vi "首页.vi"() -> ()   [LabVIEW 2016]
uses:
  <vilib>/Utility/miscctls.llb/LVPointTypeDef.ctl
  <vilib>/Utility/sysdir.llb/System Directory Type.ctl
  <vilib>/addons/database/_DB Variant To Data/Database Variant To Data.xnode
  PLC/PLC.lvlib
panel:
  out "小项目框 10":T1(xcontrol)
  out "小项目框 9":T1(xcontrol)
  out "小项目框 4":T1(xcontrol)
  out "小项目框 3":T1(xcontrol)
  out "小项目框 2":T1(xcontrol)
  out "小项目框 8":T1(xcontrol)
  out "小项目框 7":T1(xcontrol)
  out "小项目框 6":T1(xcontrol)
  out "小项目框 5":T1(xcontrol)
  out "小项目框":T1(xcontrol)
  out "湿度":string="75.5 %"
  out "室温":string="25.8 ℃"
  # "湿度:"
  # "室温:"
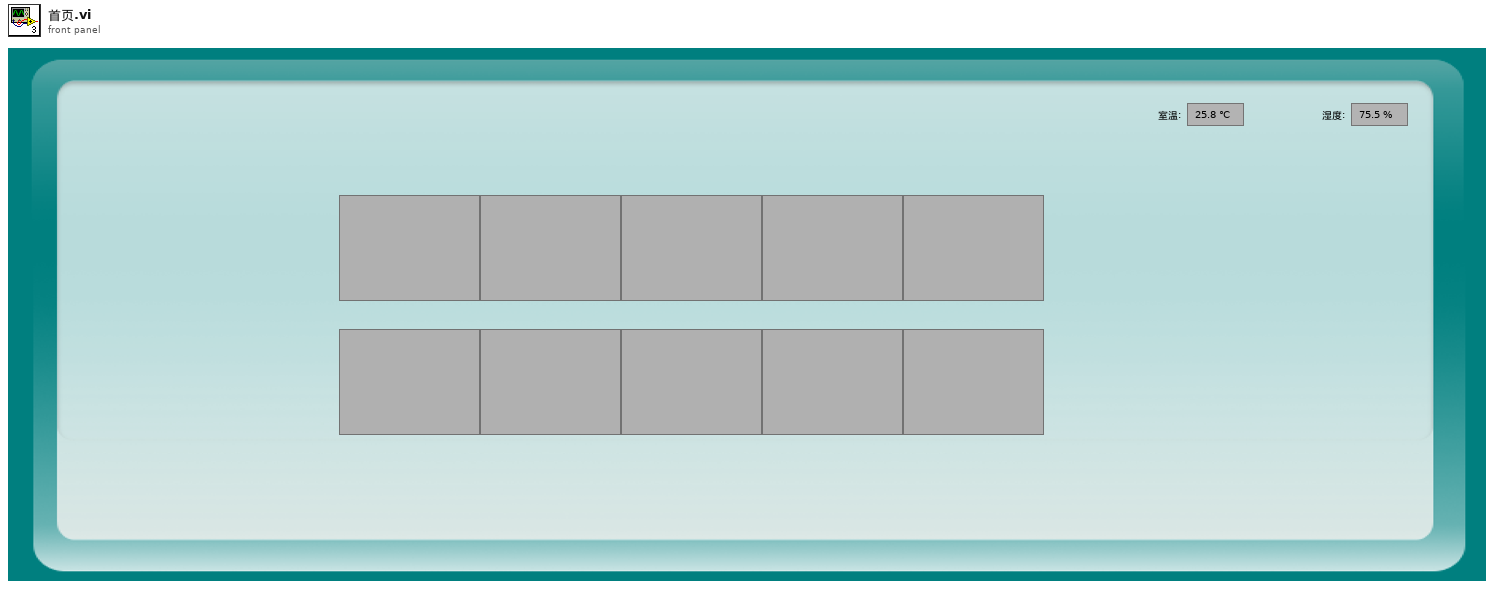
[diagram p1: front panel]
types:
  T1 = cluster{"中文项目名称":string, "英文项目名称":string, "单位":string, "浓度值":sgl, "精度":sgl}
  T2 = typedef "System Directory Type.ctl" = i32
  T3 = typedef "LVPointTypeDef.ctl" = cluster{"Horizontal":i16, "Vertical":i16}
  T4 = cluster{"AD0":sgl, "AD1":sgl, "AD2":sgl, "AD3":sgl, "AD4":sgl, "AD5":sgl}
  T5 = typedef "LVDateTimeRec.ctl" = cluster{"秒数的小数部分":dbl, "秒":i32, "分":i32, "时":i32, "日":i32, "月":i32, "年":i32, "天数（周）":i32, "天数（年）":i32, "DST":i32}
  T6 = cluster{"seconds since 1Jan1904":timestamp, "AD0":sgl, "单位":u16}
  T7 = cluster{"seconds since 1Jan1904":timestamp, "AD1":sgl, "单位":u16}
  T8 = cluster{"时间标识":timestamp, "监测值":sgl, "单位":string}
  T9 = cluster{"中文项目名称":string, "英文项目名称":string, "单位":string, "浓度值":sgl, "浓度值 2":sgl}
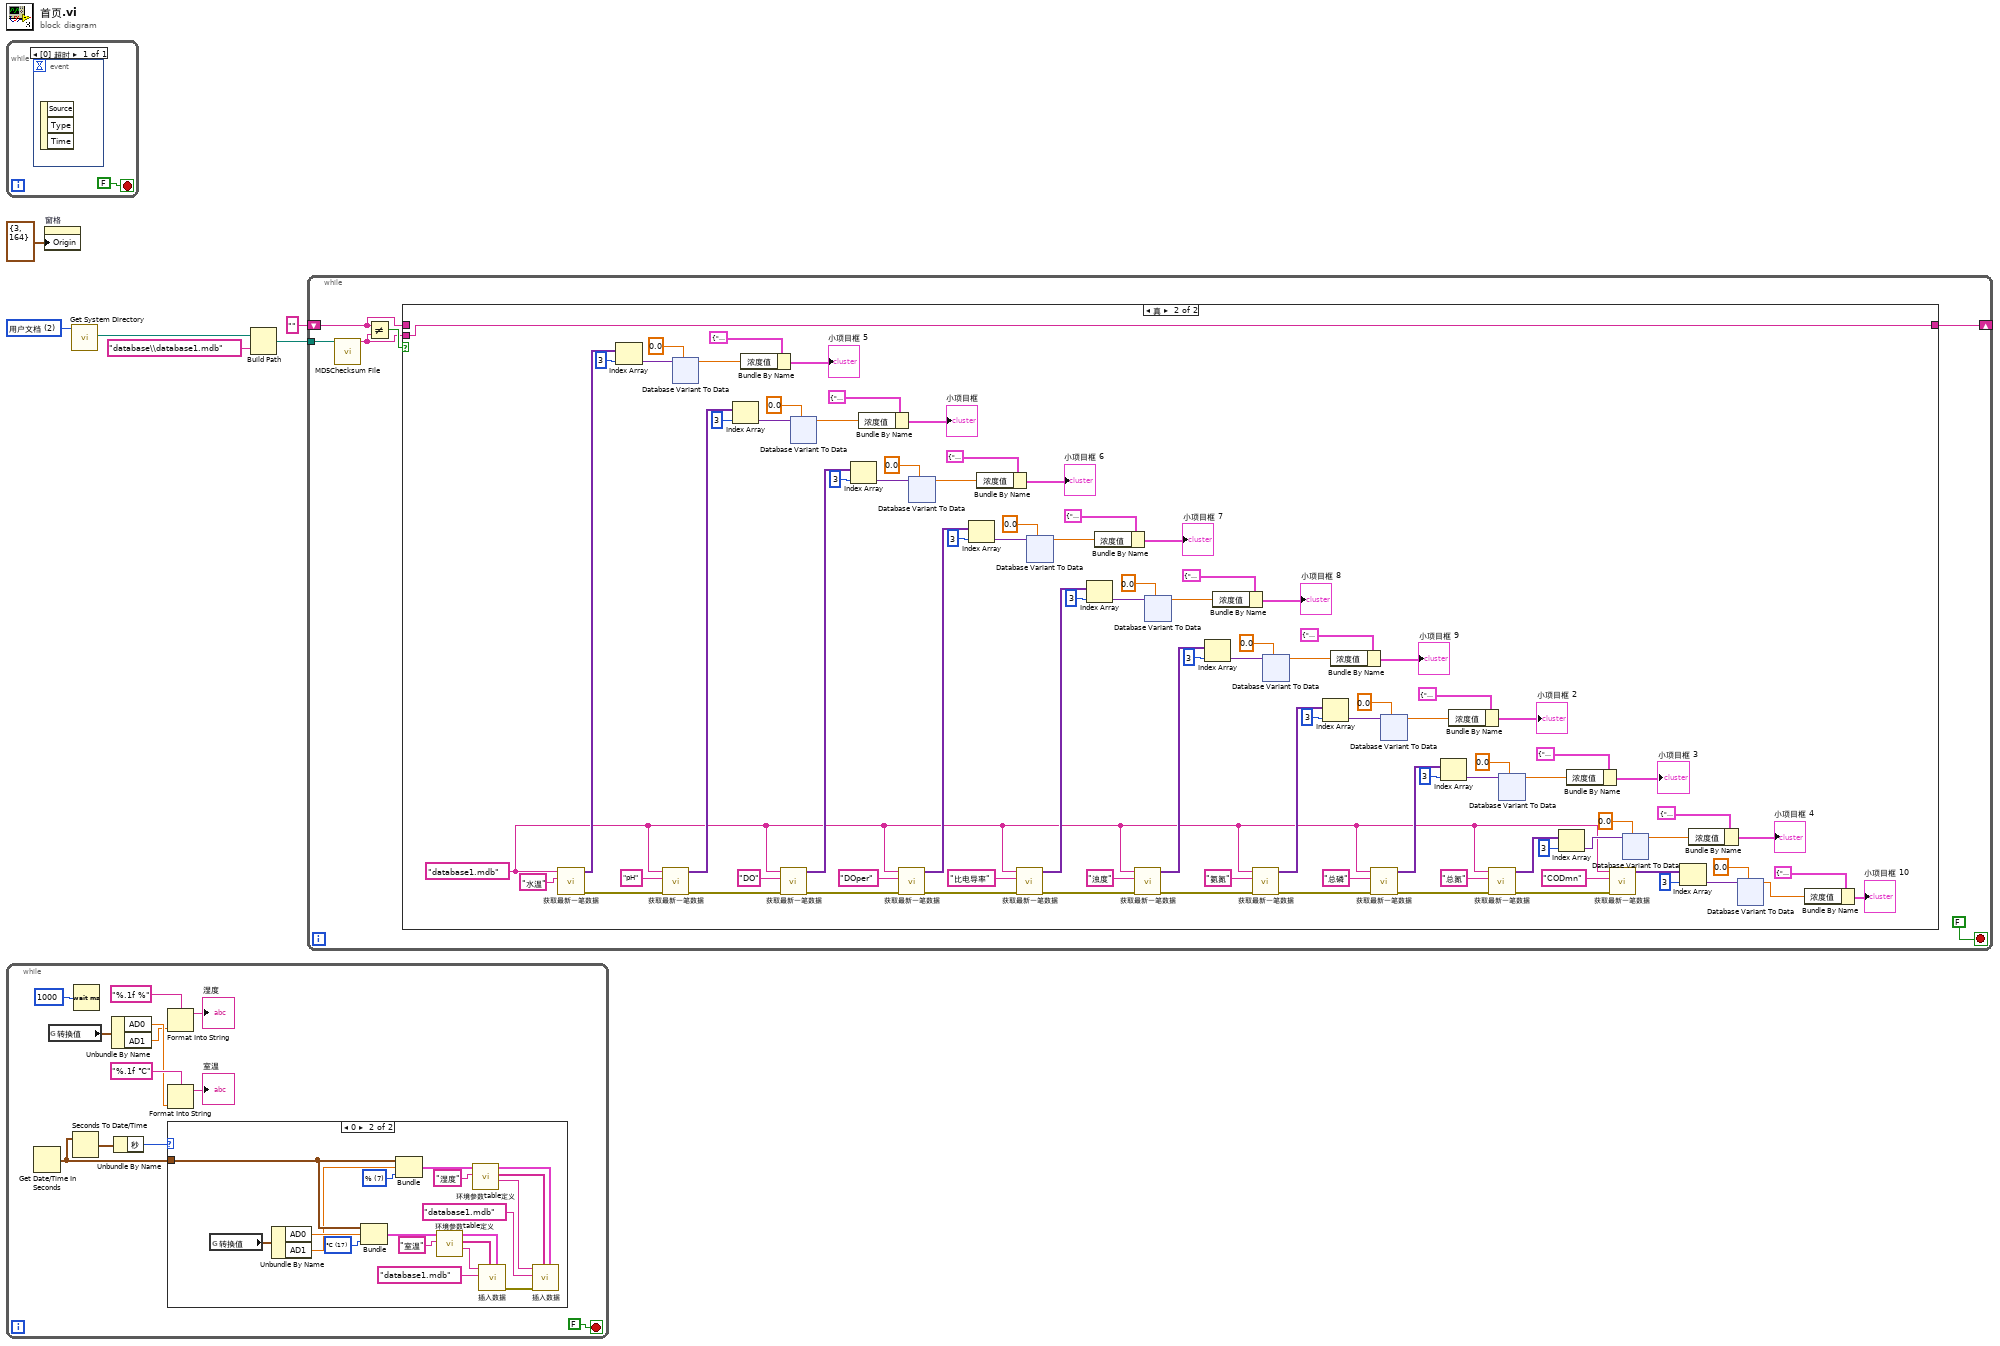
[diagram p0: block diagram]
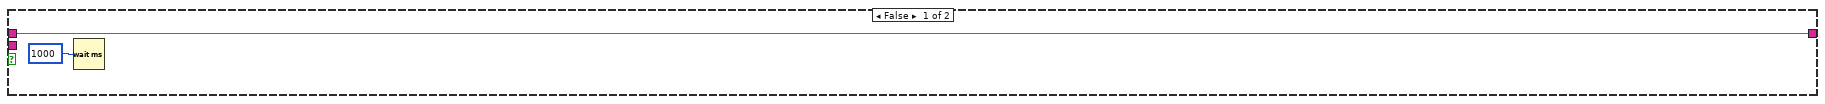
[diagram p2: hidden frame]
diagram:
  w5 = T2 2 items=["用户目录"=0, "用户桌面"=1, "用户文档"=2, "用户应用程序数据"=3, "用户设置"=4, "用户临时目录"=5, "公共文档"=6, "公共应用程序数据"=7, "公共设置"=8, "公共缓存"=13, "系统核心库"=9, "系统安装库"=10, "应用程序文件"=11, "启动盘根目录"=12] ("system directory type")
  n1 = while {
    stop <- FALSE stop-if-true
    n2 = event shown="[0] 超时" {
      selector: _ -> [_]
      dyn-events: _ -> [_]
      timeout: _ -> [_]
      event Timeout {
        n3 = event-data() -> ()  [unwired: 1 in, 3 out]
      }
    }
  }
  n4 = while {
    stop <- FALSE stop-if-true
    n5 = Get Date/Time In Seconds() -> (seconds since 1Jan1904=w10:timestamp)
    n6 = global read "采配水全局变量.vi" "转换值"() -> (w17:T4)
    n7 = Seconds To Date/Time(time stamp (now)=w10) -> (date time rec=w9:T5)  [unwired: 1 in]
    n8 = Wait (ms)(milliseconds to wait=u32 1000 ("等待时间（毫秒）")) -> ()  [unwired: 1 out]
    n9 = Unbundle By Name(w17) -> ("AD0"=w12:sgl, "AD1"=w11:sgl)
    n10 = Unbundle By Name(w9) -> ("秒"=w8:i32)
    n11 = Format Into String(format string="%.1f %" ("格式字符串"), w11) -> (resulting string=→"湿度":string)  [unwired: 2 in, 1 out]
    n12 = Format Into String(format string="%.1f ℃" ("格式字符串"), w12) -> (resulting string=→"室温":string)  [unwired: 2 in, 1 out]
    n13 = case shown="0" w8 {
      tunnel: w10 -> [_ w25]
      frame Default {
      }
      frame 0 {
        w23 = u16 7 items=["ug/L", "mg/L", "ppm", "mg/m3", "cm", "ppb", "ug/m3", "%", "nmol/mol", "umol/mol", "MPN/L", "MPN/100ml", "ng/m3", "NTU", "无量纲", "ms/cm", "us/cm", "℃"] ("单位")
        w26 = u16 17 items=["ug/L", "mg/L", "ppm", "mg/m3", "cm", "ppb", "ug/m3", "%", "nmol/mol", "umol/mol", "MPN/L", "MPN/100ml", "ng/m3", "NTU", "无量纲", "ms/cm", "us/cm", "℃"] ("单位")
        n14 = global read "采配水全局变量.vi" "转换值"() -> (w34:T4)
        n15 = Unbundle By Name(w34) -> ("AD0"=w28:sgl, "AD1"=w24:sgl)
        n16 = Bundle("seconds since 1Jan1904"=w25, "AD0"=w28, "单位"=w26) -> (w27:T6)  [unwired: 1 in]
        n17 = Bundle("seconds since 1Jan1904"=w25, "AD1"=w24, "单位"=w23) -> (w22:T7)  [unwired: 1 in]
        n18 = call "环境参数table定义.vi"("table 输入"="室温", "data"=w27) -> ("table 输出"=w35:string, "columns"=w36:string[], "data输出"=w37:T8)  [unwired: 7 in]
        n19 = call "环境参数table定义.vi"("table 输入"="湿度", "data"=w22) -> ("table 输出"=w33:string, "columns"=w32:string[], "data输出"=w31:T8)  [unwired: 7 in]
        n20 = call "插入数据.vi"("data"=w37, "columns"=w36, "database"="database1.mdb", "table"=w35) -> ("error out"=w29:errorcluster)  [unwired: 7 in]
        n21 = call "插入数据.vi"("data"=w31, "columns"=w32, "error in (no error)"=w29, "database"="database1.mdb", "table"=w33) -> ()  [unwired: 6 in, 1 out]
      }
    }
  }
  n22 = property on="窗格" class="Pane"("Origin"=T3 {"Horizontal"=3, "Vertical"=164} ("原点")) -> ()  [unwired: 2 in, 2 out]
  n23 = call <vilib>:"Get System Directory.vi"("system directory type"=w5) -> ("system directory"=w4:path)  [unwired: 10 in]
  n24 = Build Path(base path=w4, name or relative path="database\\database1.mdb" ("名称或相对路径")) -> (appended path=w2:path)
  n25 = while {
    tunnel: w2 -> [w44]
    shift-right: [w41] -> _
    shift-left: "" ("MD5 message-digest") -> [w40]
    stop <- FALSE stop-if-true
    n26 = call <vilib>:"MD5Checksum File.vi"("Path"=w44) -> ("MD5 message-digest"=w42:string)  [unwired: 9 in, 1 out]
    n27 = Not Equal?(x=w40, y=w42) -> (x != y?=w43:bool)
    n28 = case shown="真" w43 {
      tunnel: w42 -> [_ w137]
      tunnel: [w46 w137] -> w41
      tunnel: w40 -> [w46 _]
      frame False {
        n29 = Wait (ms)(milliseconds to wait=u32 1000 ("等待时间（毫秒）")) -> ()  [unwired: 1 out]
      }
      frame True {
        w55 = "database1.mdb" ("名称或相对路径")
        n30 = call "获取最新一笔数据.vi"("table"="水温", "database"=w55) -> ("error out"=w101:errorcluster, "子数组"=w67:variant[])  [unwired: 8 in]
        n31 = Index Array(array=w67, index=3 ("索引")) -> (element=w90:variant)
        n32 = call "获取最新一笔数据.vi"("error in (no error)"=w101, "table"="pH", "database"=w55) -> ("error out"=w100:errorcluster, "子数组"=w126:variant[])  [unwired: 7 in]
        n33 = xnode "Database Variant To Data"("database variant"=w90, "type"=0.0) -> ("data"=w92:dbl)  [unwired: 1 in, 1 out]
        n34 = Index Array(array=w126, index=3 ("索引")) -> (element=w109:variant)
        n35 = Bundle By Name(cluster=T9 {"中文项目名称"="水温", "英文项目名称"="T", "单位"="℃", "浓度值"=0.0, "浓度值 2"=2.0} ("小项目框 9"), "浓度值"=w92) -> (→"小项目框 5":T9)
        n36 = call "获取最新一笔数据.vi"("error in (no error)"=w100, "table"="DO", "database"=w55) -> ("error out"=w98:errorcluster, "子数组"=w66:variant[])  [unwired: 7 in]
        n37 = xnode "Database Variant To Data"("database variant"=w109, "type"=0.0) -> ("data"=w107:dbl)  [unwired: 1 in, 1 out]
        n38 = Index Array(array=w66, index=3 ("索引")) -> (element=w85:variant)
        n39 = Bundle By Name(cluster=T9 {"中文项目名称"="酸碱度", "英文项目名称"="pH", "单位"="", "浓度值"=0.0, "浓度值 2"=2.0} ("小项目框 9"), "浓度值"=w107) -> (→"小项目框":T9)
        n40 = call "获取最新一笔数据.vi"("error in (no error)"=w98, "table"="DOper", "database"=w55) -> ("error out"=w96:errorcluster, "子数组"=w65:variant[])  [unwired: 7 in]
        n41 = xnode "Database Variant To Data"("database variant"=w85, "type"=0.0) -> ("data"=w83:dbl)  [unwired: 1 in, 1 out]
        n42 = Index Array(array=w65, index=3 ("索引")) -> (element=w80:variant)
        n43 = Bundle By Name(cluster=T9 {"中文项目名称"="溶解氧", "英文项目名称"="DO", "单位"="mg/L", "浓度值"=0.0, "浓度值 2"=2.0} ("小项目框 9"), "浓度值"=w83) -> (→"小项目框 6":T9)
        n44 = call "获取最新一笔数据.vi"("error in (no error)"=w96, "table"="比电导率", "database"=w55) -> ("error out"=w94:errorcluster, "子数组"=w64:variant[])  [unwired: 7 in]
        n45 = xnode "Database Variant To Data"("database variant"=w80, "type"=0.0) -> ("data"=w82:dbl)  [unwired: 1 in, 1 out]
        n46 = Index Array(array=w64, index=3 ("索引")) -> (element=w75:variant)
        n47 = Bundle By Name(cluster=T9 {"中文项目名称"="溶解氧%", "英文项目名称"="DO%", "单位"="%", "浓度值"=0.0, "浓度值 2"=2.0} ("小项目框 9"), "浓度值"=w82) -> (→"小项目框 7":T9)
        n48 = call "获取最新一笔数据.vi"("error in (no error)"=w94, "table"="浊度", "database"=w55) -> ("error out"=w93:errorcluster, "子数组"=w63:variant[])  [unwired: 7 in]
        n49 = xnode "Database Variant To Data"("database variant"=w75, "type"=0.0) -> ("data"=w73:dbl)  [unwired: 1 in, 1 out]
        n50 = Index Array(array=w63, index=3 ("索引")) -> (element=w70:variant)
        n51 = Bundle By Name(cluster=T9 {"中文项目名称"="电导率", "英文项目名称"="Cond", "单位"="uS/cm", "浓度值"=0.0, "浓度值 2"=2.0} ("小项目框 9"), "浓度值"=w73) -> (→"小项目框 8":T9)
        n52 = call "获取最新一笔数据.vi"("error in (no error)"=w93, "table"="氨氮", "database"=w55) -> ("error out"=w135:errorcluster, "子数组"=w121:variant[])  [unwired: 7 in]
        n53 = xnode "Database Variant To Data"("database variant"=w70, "type"=0.0) -> ("data"=w72:dbl)  [unwired: 1 in, 1 out]
        n54 = Index Array(array=w121, index=3 ("索引")) -> (element=w115:variant)
        n55 = Bundle By Name(cluster=T9 {"中文项目名称"="浊度", "英文项目名称"="Turb", "单位"="NTU", "浓度值"=0.0, "浓度值 2"=2.0} ("小项目框 9"), "浓度值"=w72) -> (→"小项目框 9":T9)
        n56 = call "获取最新一笔数据.vi"("error in (no error)"=w135, "table"="总磷", "database"=w55) -> ("error out"=w103:errorcluster, "子数组"=w116:variant[])  [unwired: 7 in]
        n57 = xnode "Database Variant To Data"("database variant"=w115, "type"=0.0) -> ("data"=w113:dbl)  [unwired: 1 in, 1 out]
        n58 = Index Array(array=w116, index=3 ("索引")) -> (element=w112:variant)
        n59 = Bundle By Name(cluster=T9 {"中文项目名称"="氨氮", "英文项目名称"="NH3-N", "单位"="mg/L", "浓度值"=0.0, "浓度值 2"=3.0} ("小项目框 9"), "浓度值"=w113) -> (→"小项目框 2":T9)
        n60 = call "获取最新一笔数据.vi"("error in (no error)"=w103, "table"="总氮", "database"=w55) -> ("error out"=w56:errorcluster, "子数组"=w129:variant[])  [unwired: 7 in]
        n61 = xnode "Database Variant To Data"("database variant"=w112, "type"=0.0) -> ("data"=w110:dbl)  [unwired: 1 in, 1 out]
        n62 = Index Array(array=w129, index=3 ("索引")) -> (element=w106:variant)
        n63 = Bundle By Name(cluster=T9 {"中文项目名称"="总磷", "英文项目名称"="TP", "单位"="mg/L", "浓度值"=0.0, "浓度值 2"=3.0} ("小项目框 9"), "浓度值"=w110) -> (→"小项目框 3":T9)
        n64 = call "获取最新一笔数据.vi"("error in (no error)"=w56, "table"="CODmn", "database"=w55) -> ("子数组"=w53:variant[])  [unwired: 7 in, 1 out]
        n65 = xnode "Database Variant To Data"("database variant"=w106, "type"=0.0) -> ("data"=w104:dbl)  [unwired: 1 in, 1 out]
        n66 = Index Array(array=w53, index=3 ("索引")) -> (element=w51:variant)
        n67 = Bundle By Name(cluster=T9 {"中文项目名称"="总氮", "英文项目名称"="TN", "单位"="mg/L", "浓度值"=0.0, "浓度值 2"=3.0} ("小项目框 9"), "浓度值"=w104) -> (→"小项目框 4":T9)
        n68 = xnode "Database Variant To Data"("database variant"=w51, "type"=0.0) -> ("data"=w48:dbl)  [unwired: 1 in, 1 out]
        n69 = Bundle By Name(cluster=T9 {"中文项目名称"="高锰酸盐指数", "英文项目名称"="CODmn", "单位"="mg/L", "浓度值"=0.0, "浓度值 2"=2.0} ("小项目框 9"), "浓度值"=w48) -> (→"小项目框 10":T9)
      }
    }
  }
